vi "manualChannelConfiguration.vi"(8 "error in":T1) -> (0 "error out":T1, 3 "storage paths":string[](array[string]))   [LabVIEW 2016]
doc: "A pop up window will appear when this VI is called. It shows the current channel configuration. If you want to change the configuration, enter the desired values into the channel-parameters-cluster and press \"apply changes\". The changes can be checked in the table beneath. Furthermore it is possible to define a storage path for each channel. A string array with fourteen string elements containing the set storage paths will be provided by the VI. The storage path of channel 1 will be stored in the array at index 1."
uses:
  Controls/Channel-Source_Selection.ctl
  Controls/Trigger_Selection.ctl
  Controls/Error_Out.ctl
  Controls/Channel_Parameters.ctl
  Controls/Channel_Selection.ctl
  Controls/Average_Selection.ctl
panel:
  in  "Array":string[](array[string])=["Storage path", "", "", "", "", "", "", "", "", "", "", "", "", "", ""]
  in  "storage path":string
  in  "stop":bool
  in  "apply changes":bool
  in  "Channel Parameters Cluster":T2={"Channel"=1, "Source"=1, "Average"=1, "SampleTime [us]"=5000.0, "Trigger"=1} {"Trigger" items=["[read only]"=-2147483648, "Disabled"=0, "Scanner"=1, "Permanent"=2, "Spectroscopy 1"=3, "Spectroscopy 2"=4, "Spectroscopy 3"=5, "Calibration"=6, "Trigger"=7, "Every"=8, "Command"=9, "2nd Pass"=13, "Step Scan"=16]; "Average" items=["[read only]"=-2147483648, "no"=0, "yes"=1]; "Source" items=["[read only]"=-2147483648, "ADC 1"=0, "ADC 2"=1, "ADC 3"=2, "ADC 4"=3, "ADC 5"=4, "ADC 6"=5, "HF 1 Out"=7, "HF 1 df"=8, "z out"=9, "HF 1"=12, "HF 1 Ampl."=13, "HF 1 Phase"=14, "LF LockIn Ampl"=16, "LF LockIn Phase"=17, "z out inv"=18, "counter"=23, "Crosslink 1"=29, "Crosslink 2"=30, "Pos X"=31, "Pos Y"=32]; "Channel" items=["Channel 0", "Channel 1", "Channel 2", "Channel 3", "Channel 4", "Channel 5", "Channel 6", "Channel 7", "Channel 8", "Channel 9", "Channel 10", "Channel 11", "Channel 12", "Channel 13"]}
  out "Trigger":T6 items=["[read only]"=-2147483648, "Disabled"=0, "Scanner"=1, "Permanent"=2, "Spectroscopy 1"=3, "Spectroscopy 2"=4, "Spectroscopy 3"=5, "Calibration"=6, "Trigger"=7, "Every"=8, "Command"=9, "2nd Pass"=13, "Step Scan"=16]
  out "Source":T4 items=["[read only]"=-2147483648, "ADC 1"=0, "ADC 2"=1, "ADC 3"=2, "ADC 4"=3, "ADC 5"=4, "ADC 6"=5, "HF 1 Out"=7, "HF 1 df"=8, "z out"=9, "HF 1"=12, "HF 1 Ampl."=13, "HF 1 Phase"=14, "LF LockIn Ampl"=16, "LF LockIn Phase"=17, "z out inv"=18, "counter"=23, "Crosslink 1"=29, "Crosslink 2"=30, "Pos X"=31, "Pos Y"=32]
  out "output array":string[][](table)
  # "Note: Applied Changes might not be reflected within Daisy!"
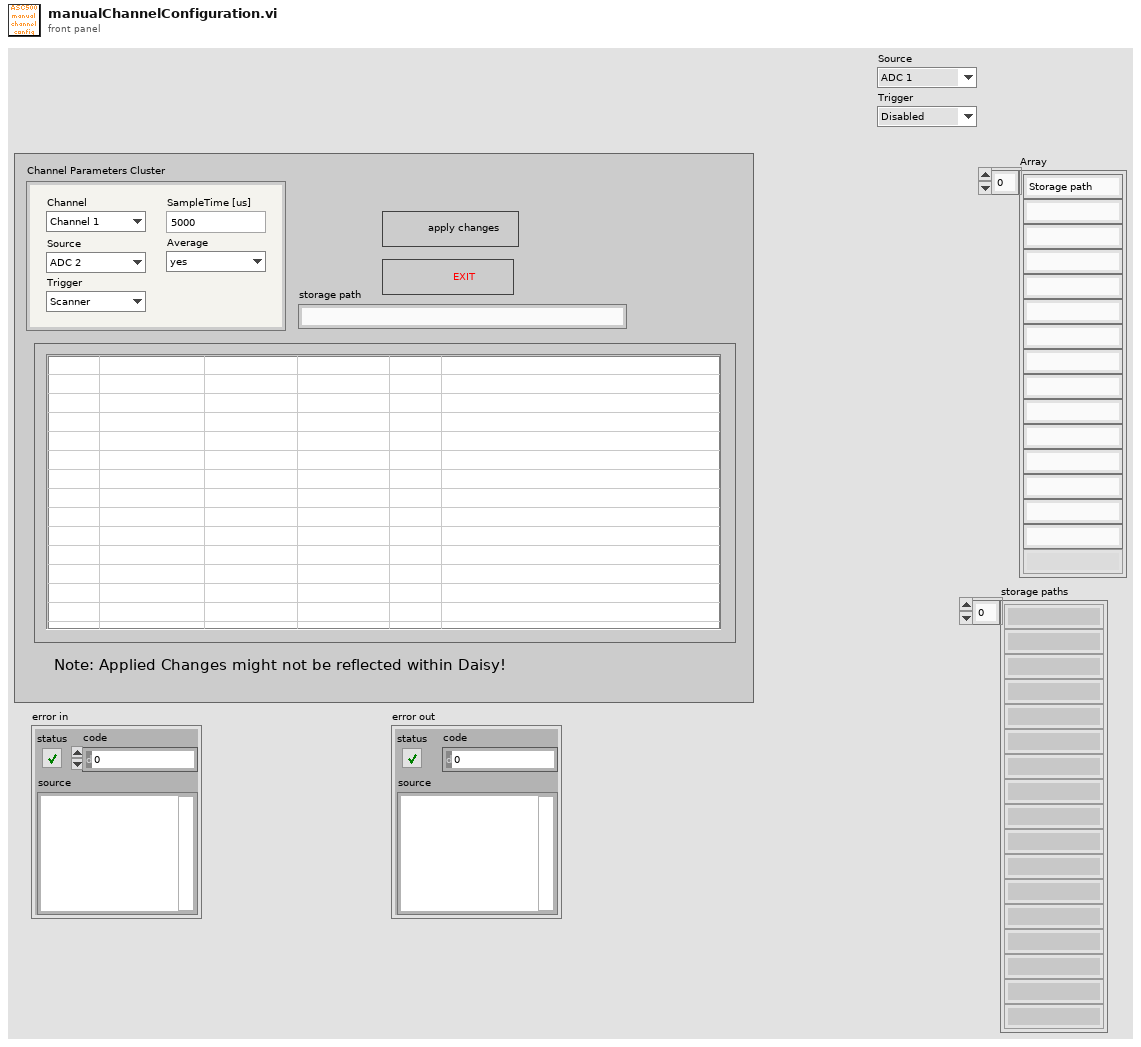
[diagram p1: front panel]
types:
  T1 = typedef "Error_Out.ctl" = errorcluster
  T2 = typedef "Channel_Parameters.ctl" = cluster{"Channel":T3, "Source":T4, "Average":T5, "SampleTime [us]":sgl, "Trigger":T6}
  T3 = typedef "Channel_Selection.ctl" = i32
  T4 = typedef "Channel-Source_Selection.ctl" = i32
  T5 = typedef "Average_Selection.ctl" = i32
  T6 = typedef "Trigger_Selection.ctl" = i32
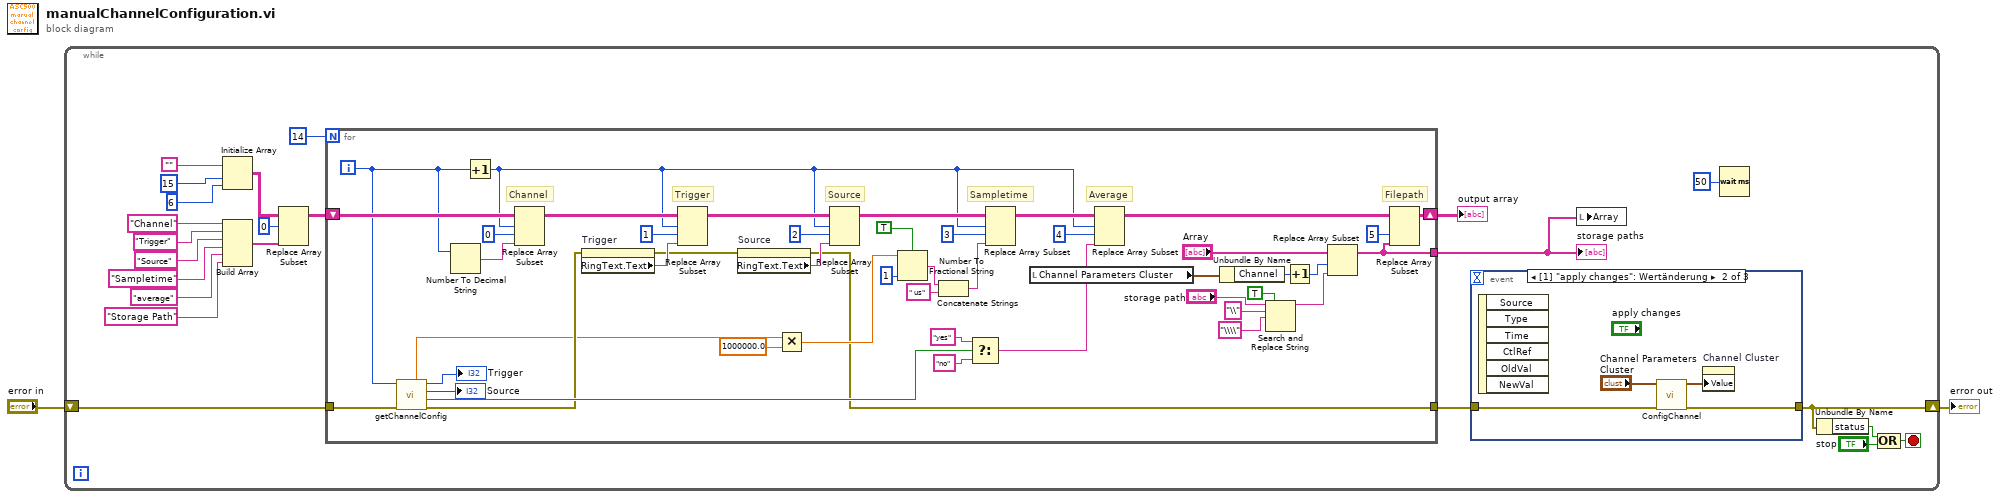
[diagram p0: block diagram]
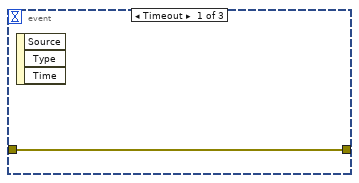
[diagram p2: hidden frame]
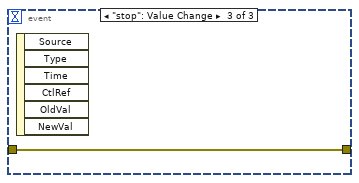
[diagram p3: hidden frame]
diagram:
  n1 = while {
    shift-right: [w10] -> w2
    shift-left: "error in" -> [w11]
    stop <- w9 stop-if-true
    n2 = Initialize Array("" ("String"), 15 ("dimension size"), 6 ("dimension size 2")) -> (w23:string[][])
    n3 = Build Array("Channel" ("String 3"), "Trigger" ("String 3"), "Source" ("String 3"), "Sampletime" ("String 3"), "average" ("String 3"), "Storage Path" ("element")) -> (w25:string[])
    n4 = Replace Array Subset(array=w23, new element=w25, index (row)=0) -> (w14:string[][])  [unwired: 1 in]
    n5 = for {
      N: 14 -> [_]
      shift-right: [w45] -> w4
      shift-left: w14 -> [w73]
      tunnel: w11 -> [w64]
      tunnel: [w51] -> w12
      tunnel: [w39] -> w3
      i -> [w56]
      # "Filepath"
      # "Average"
      # "Source"
      # "Sampletime"
      # "Trigger"
      # "Channel"
      n6 = call "getChannelConfig.vi"("error in"=w64, "Channel"=w56) -> ("error out"=w52:T1, "Averaging?"=w70:bool, "source"=→"Source":i32, "trigger"=→"Trigger":i32, "smpTime"=w42:dbl)  [unwired: 5 in]
      n7 = Number To Decimal String(number=w56) -> (decimal integer string=w76:string)  [unwired: 1 in]
      n8 = Increment(x=w56) -> (x+1=w47:i32)
      n9 = Replace Array Subset(array=w73, new element=w76, index (row)=w47, index (col)=0 ("disabled index (col)")) -> (w63:string[][])
      n10 = property on="Trigger" class="Ring (strikt)"(error in=w52) -> (error out=w53:errorcluster, "RingText.Text"=w66:string)  [unwired: 1 in, 1 out]
      n11 = Replace Array Subset(array=w63, new element=w66, index (row)=w47, index (col)=1 ("disabled index (col)")) -> (w62:string[][])
      n12 = property on="Source" class="Ring (strikt)"(error in=w53) -> (error out=w51:errorcluster, "RingText.Text"=w65:string)  [unwired: 1 in, 1 out]
      n13 = Multiply(x=w42, y=1000000.0) -> (x*y=w58:dbl)
      n14 = Replace Array Subset(array=w62, new element=w65, index (row)=w47, index (col)=2 ("disabled index (col)")) -> (w61:string[][])
      n15 = Number To Fractional String(use system decimal point (T)=TRUE, number=w58, precision (6)=i16 1) -> (F-format string=w50:string)  [unwired: 1 in]
      n16 = Concatenate Strings(w50, " us" ("string")) -> (w48:string)
      n17 = Select(t="yes", s=w70, f="no") -> (s? t:f=w67:string)
      n18 = Replace Array Subset(array=w61, new element=w48, index (row)=w47, index (col)=3 ("disabled index (col)")) -> (w60:string[][])
      n19 = local read "Channel Parameters Cluster"() -> (w46:T2)
      n20 = Replace Array Subset(array=w60, new element=w67, index (row)=w47, index (col)=4 ("disabled index (col)")) -> (w40:string[][])
      n21 = Unbundle By Name(w46) -> ("Channel"=w44:T3)
      n22 = Search and Replace String(replace all?=TRUE ("replace all? (F)"), input string="storage path", search string="\\", replace string="\\\\" ("replace string (\"\")")) -> (result string=w34:string)  [unwired: 4 in, 3 out]
      n23 = Increment(x=w44) -> (x+1=w41:T3)
      n24 = Replace Array Subset(array="Array", new element=w34, index=w41) -> (w39:string[])
      n25 = Replace Array Subset(array=w40, new element=w39, index (col)=5 ("disabled index (col)")) -> (w45:string[][])  [unwired: 1 in]
    }
    "output array" <- w4
    "storage paths" <- w3
    n26 = event shown="[1] \"apply changes\": Wertänderung" {
      selector: _ -> [_ _ _]
      dyn-events: _ -> [_ _ _]
      timeout: _ -> [_ _ _]
      tunnel: w12 -> [w26 w29 w31]
      tunnel: [w26 w28 w31] -> w10
      event Timeout {
        n27 = event-data() -> ()  [unwired: 1 in, 3 out]
      }
      event "apply changes": Value Change {
        n28 = event-data() -> ()  [unwired: 1 in, 6 out]
        n29 = call "ConfigChannel.vi"("error in"=w29, "Channel Cluster"="Channel Parameters Cluster") -> ("error out"=w28:T1, "Output Cluster"=w27:T2)  [unwired: 8 in]
        n30 = property on="Channel Cluster" class="Cluster (strikt)"("Value"=w27) -> ()  [unwired: 2 in, 2 out]
      }
      event "stop": Value Change {
        n31 = event-data() -> ()  [unwired: 1 in, 6 out]
      }
    }
    n32 = local write "Array"(w3) -> ()
    n33 = Wait (ms)(milliseconds to wait=u32 50) -> ()  [unwired: 1 out]
    n34 = Unbundle By Name(w10) -> ("status"=w8:bool)
    n35 = Compound Arithmetic op=OR(w8, "stop") -> (w9:bool)
  }
  "error out" <- w2
